vi "Get Category.vi"(8 "error in (no error)":errorcluster, 11 "Scan Engine editor node in":refnum<class "Scan Engine editor node.lvclass">) -> (0 "error out":errorcluster, 2 "Category":string, 3 "Scan Engine editor node out":refnum<class "Scan Engine editor node.lvclass">)   [LabVIEW 2015, in "Scan Engine editor node.lvclass"]
uses:
  Scan Engine editor node.lvclass
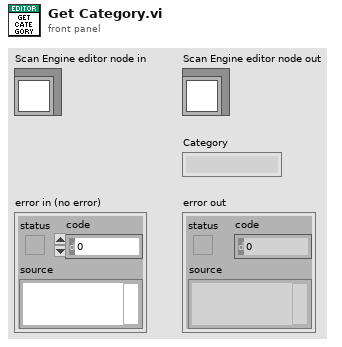
[diagram p1: front panel]
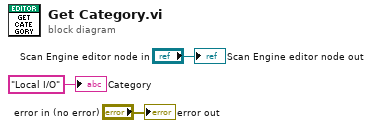
[diagram p0: block diagram]
diagram:
  "error out" <- "error in (no error)"
  "Scan Engine editor node out" <- "Scan Engine editor node in"
  "Category" <- "Local I/O" ("Category")
